vi "GetTerms3.vi"(0 "XRef":T10, 1 "State In":T9) -> (14 "Terms":T1)   [LabVIEW 2013, in "Write Exception Property.xnode"]
doc: "This ability VI is used to describe your terminals to LabVIEW. Terms is an array of clusters describing the XNode's terminals.\n ID: A unique string identifying the terminal.\n Name: The name of the terminal visible to the user. Remember to localize it.\n Type: The data type of the terminal (as a Variant). The data put in the variant will be used as the default for the input terminal if it's left unwired.\n Bounds: A rectangle defining the bounds of the terminal relative to the bounds of the XNode. The bounds must be within the bounds of the XNode, and for whiskers to draw properly, they must be flush with at least one side of the XNode.\n Input?: Indicates whether or not this terminals is an input.\n Required?: Indicates whether the user must wire this terminal for the XNode to not be broken. Ignored on outputs.\n Recommended?: Indicates whether the terminal is recommended.\n Hidden?: Indicates whether the terminal is hidden. When a terminal is hidden, it cannot be wired to via user interaction or scripting. However, if it is already wired to when the hidden flag is changed to true, it will remain wired.\n Adaptive?: Indicates that the term should change to match the type of its source if it is wired.\n Direction?: Indicates what direction the wire stub should point. Choose auto to let LV decide based on the terms bounds being on the nodes edge.\n \n The IDs are used by LabVIEW to keep track of your terminals. When you respecify your terminals, LabVIEW can tell whther terminals are new, deleted, or moved by the unique IDs. The order is irrelevant. If you move a terminal, then any wire connected to it will move with it.\n \n If you want to update your terminals, you should return the UpdateTerms reply in one of your ability VIs.\n\nDefault behavior: None.\n\nThis ability does not provide UI and OS messages are not handled.\n\n\n-------------\nBrian Hoover (Hooovahh)\n\nProduct Name: Variant Repository\nPackage File Name: lava_lib_variant_repository\nPackage Version: 1.0.1.11\nMinimum LabVIEW Version: 11.0"
uses:
  Write Exception Property.xnode
  <vilib>/XNodeSupport/XNodeXNodeRef.ctl
  State.ctl
  <vilib>/XNodeSupport/XNodeTerm3Array.ctl
  <vilib>/XNodeSupport/XNodeTerm3.ctl
  <vilib>/XNodeSupport/XNodeString.ctl
  <vilib>/XNodeSupport/XNodeVariant.ctl
  <vilib>/XNodeSupport/XNodeRect32.ctl
  <vilib>/XNodeSupport/XNodeInt.ctl
  <vilib>/XNodeSupport/XNodeBool.ctl
  <vilib>/XNodeSupport/XNodeTermDirection.ctl
  failure.ctl
  <vilib>/XNodeSupport/NI_XNodeSupport.lvlib
  failure.lvlib
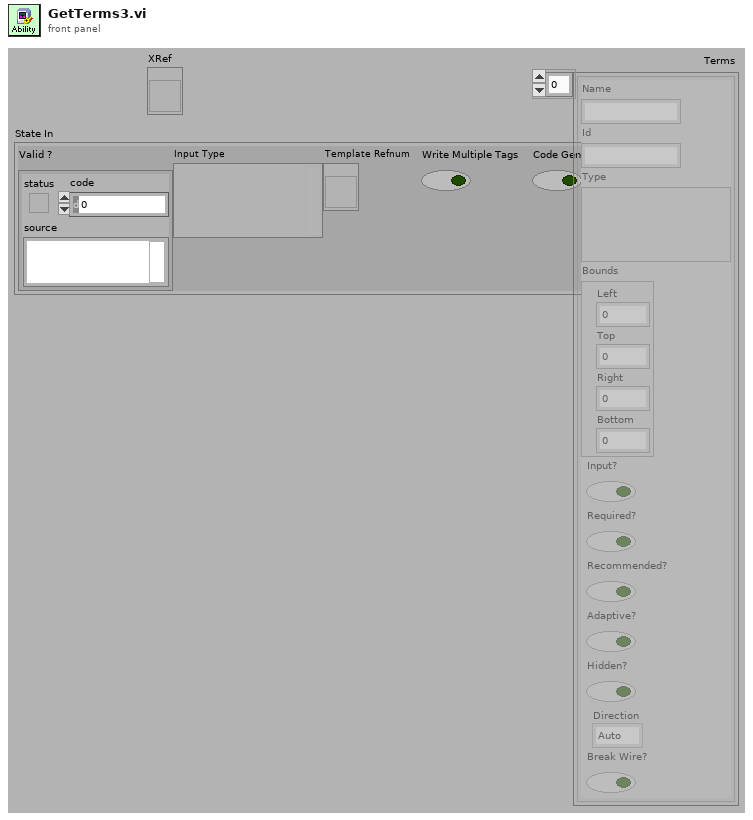
[diagram p1: front panel]
types:
  T1 = typedef "NI_XNodeSupport.lvlib/XNodeTerm3Array.ctl" = T2[]
  T2 = typedef "NI_XNodeSupport.lvlib/XNodeTerm3.ctl" = cluster{"Name":T3, "Id":T3, "Type":T4, "Bounds":T5, "Input?":T7, "Required?":T7, "Recommended?":T7, "Adaptive?":T7, "Hidden?":T7, "Direction":T8, "Break Wire?":T7}
  T3 = typedef "NI_XNodeSupport.lvlib/XNodeString.ctl" = string
  T4 = typedef "NI_XNodeSupport.lvlib/XNodeVariant.ctl" = variant
  T5 = typedef "NI_XNodeSupport.lvlib/XNodeRect32.ctl" = cluster{"Left":T6, "Top":T6, "Right":T6, "Bottom":T6}
  T6 = typedef "NI_XNodeSupport.lvlib/XNodeInt.ctl" = i32
  T7 = typedef "NI_XNodeSupport.lvlib/XNodeBool.ctl" = bool
  T8 = typedef "NI_XNodeSupport.lvlib/XNodeTermDirection.ctl" = enum32{"Auto", "Up", "Down", "Left", "Right", "Center"}
  T9 = typedef "Write Exception Property.xnode/State.ctl" = cluster{"Valid ?":errorcluster, "Input Type":variant, "Template Refnum":refnum<vi>, "Write Multiple Tags":bool, "Code Generated Once":bool}
  T10 = typedef "NI_XNodeSupport.lvlib/XNodeXNodeRef.ctl" = refnum<vi>
  T11 = typedef "failure.lvlib/failure.ctl" = cluster{"code":i32, "properties":variant}
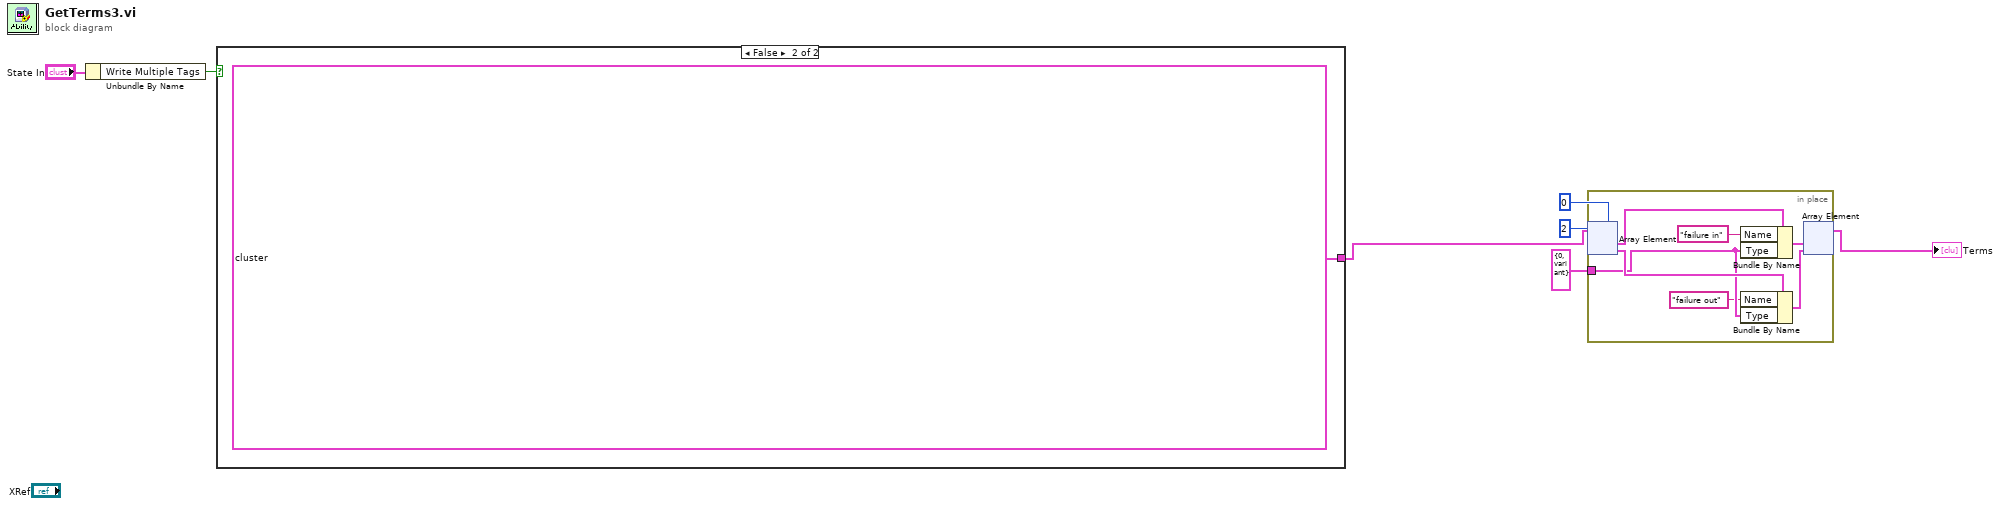
[diagram p0: block diagram]
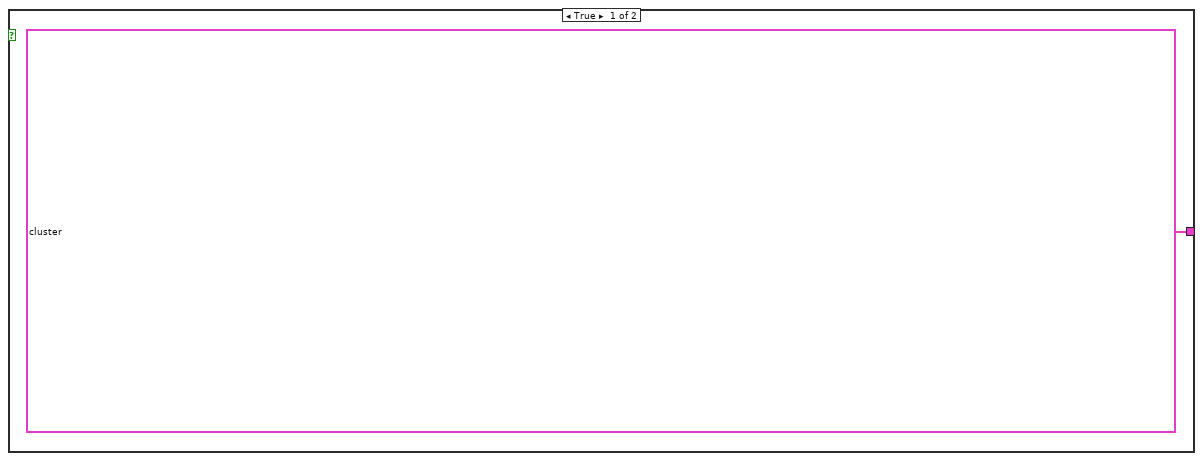
[diagram p2: hidden frame]
diagram:
  n1 = Unbundle By Name("State In") -> ("Write Multiple Tags"=w6:bool)
  n2 = case shown="False" w6 {
    tunnel: [T2[] [{"Name"="exception in", "Id"="exception in", "Type"=variant(cluster{"code":i32, "context":enum16{"developer", "user interface", "standard", "limited", "deterministic"}, "properties":variant} {"code"=0, "context"=enum."developer", "properties"=variant}), "Bounds"={"Left"=0, "Top"=0, "Right"=7, "Bottom"=7}, "Input?"=TRUE, "Required?"=TRUE, "Recommended?"=TRUE, "Adaptive?"=FALSE, "Hidden?"=FALSE, "Direction"=enum."Auto", "Break Wire?"=FALSE}, {"Name"="Tags", "Id"="Tag", "Type"=variant(string[] []), "Bounds"={"Left"=7, "Top"=0, "Right"=13, "Bottom"=16}, "Input?"=TRUE, "Required?"=TRUE, "Recommended?"=TRUE, "Adaptive?"=FALSE, "Hidden?"=FALSE, "Direction"=enum."Auto", "Break Wire?"=FALSE}, {"Name"="exception out", "Id"="exception out", "Type"=variant(cluster{"code":i32, "context":enum16{"developer", "user interface", "standard", "limited", "deterministic"}, "properties":variant} {"code"=0, "context"=enum."developer", "properties"=variant}), "Bounds"={"Left"=25, "Top"=0, "Right"=32, "Bottom"=7}, "Input?"=FALSE, "Required?"=FALSE, "Recommended?"=TRUE, "Adaptive?"=FALSE, "Hidden?"=FALSE, "Direction"=enum."Auto", "Break Wire?"=FALSE}, {"Name"="Values", "Id"="Value", "Type"=variant(variant[] []), "Bounds"={"Left"=0, "Top"=7, "Right"=7, "Bottom"=13}, "Input?"=TRUE, "Required?"=TRUE, "Recommended?"=TRUE, "Adaptive?"=FALSE, "Hidden?"=FALSE, "Direction"=enum."Auto", "Break Wire?"=FALSE}, {"Name"="failed", "Id"="failed", "Type"=variant(bool FALSE), "Bounds"={"Left"=25, "Top"=19, "Right"=32, "Bottom"=25}, "Input?"=FALSE, "Required?"=FALSE, "Recommended?"=TRUE, "Adaptive?"=FALSE, "Hidden?"=FALSE, "Direction"=enum."Auto", "Break Wire?"=FALSE}] ("Array") T2[] [{"Name"="exception in", "Id"="exception in", "Type"=variant(cluster{"code":i32, "context":enum16{"developer", "user interface", "standard", "limited", "deterministic"}, "properties":variant} {"code"=0, "context"=enum."developer", "properties"=variant}), "Bounds"={"Left"=0, "Top"=0, "Right"=7, "Bottom"=7}, "Input?"=TRUE, "Required?"=TRUE, "Recommended?"=TRUE, "Adaptive?"=FALSE, "Hidden?"=FALSE, "Direction"=enum."Auto", "Break Wire?"=FALSE}, {"Name"="Tag", "Id"="Tag", "Type"=variant(string ""), "Bounds"={"Left"=7, "Top"=0, "Right"=13, "Bottom"=16}, "Input?"=TRUE, "Required?"=FALSE, "Recommended?"=TRUE, "Adaptive?"=FALSE, "Hidden?"=FALSE, "Direction"=enum."Auto", "Break Wire?"=FALSE}, {"Name"="exception out", "Id"="exception out", "Type"=variant(cluster{"code":i32, "context":enum16{"developer", "user interface", "standard", "limited", "deterministic"}, "properties":variant} {"code"=0, "context"=enum."developer", "properties"=variant}), "Bounds"={"Left"=25, "Top"=0, "Right"=32, "Bottom"=7}, "Input?"=FALSE, "Required?"=FALSE, "Recommended?"=TRUE, "Adaptive?"=FALSE, "Hidden?"=FALSE, "Direction"=enum."Auto", "Break Wire?"=FALSE}, {"Name"="Value", "Id"="Value", "Type"=variant(variant variant), "Bounds"={"Left"=0, "Top"=7, "Right"=7, "Bottom"=13}, "Input?"=TRUE, "Required?"=TRUE, "Recommended?"=TRUE, "Adaptive?"=FALSE, "Hidden?"=FALSE, "Direction"=enum."Auto", "Break Wire?"=FALSE}, {"Name"="failed", "Id"="failed", "Type"=variant(bool FALSE), "Bounds"={"Left"=25, "Top"=19, "Right"=32, "Bottom"=25}, "Input?"=FALSE, "Required?"=FALSE, "Recommended?"=TRUE, "Adaptive?"=FALSE, "Hidden?"=FALSE, "Direction"=enum."Auto", "Break Wire?"=FALSE}] ("Array")] -> w1
    frame True {
    }
    frame False {
    }
  }
  n3 = in-place {
    in-place-border: T11 {"code"=0, "properties"=variant} ("exception") -> [w12]
    n4 = in-place-array #1(w1, 0, 2) -> (w16:T2, w13:T2)
    n5 = Bundle By Name(cluster=w16, "Name"=T3 "failure in", "Type"=w12) -> (w15:T2)
    n6 = Bundle By Name(cluster=w13, "Name"=T3 "failure out", "Type"=w12) -> (w14:T2)
    n7 = in-place-array #1(w15, w14) -> (→"Terms":T2[])  [unwired: 2 out]
  }
